vi "PH_Powermeter_BaseClass.ProcCases.vi"(0 "i ref in":refnum<vi>, 1 "selector":string, 2 "Data":T1, 3 "call cluster":T2={"Object"="", "Selector"="", "CallType"=enum."synchronous", "Async Object"="", "Async Selector"="", "Data Descriptor"="", "Data"=[], "Error #"=0, "Expire"=0}, 5 "error in":errorcluster) -> (14 "i ref out":refnum<vi>, 17 "answer cluster":T2={"Object"="", "Selector"="", "CallType"=enum."synchronous", "Async Object"="", "Async Selector"="", "Data Descriptor"="", "Data"=[], "Error #"=0, "Expire"=0}, 19 "error out":errorcluster)   [LabVIEW 2014, in "PH_Powermeter_BaseClass.lvlib"]
doc: "This method is called by a process from within the default case in the event loop. The methods of a class that are linked to events will be called from THIS method. Add your code here."
uses:
  PH_Powermeter_BaseClass.lvlib
  CS_Core/CSSystem/CoreDefs/CoreDefs.call_type.ctl
  CS_Core/BaseProcess/BaseProcess.descriptor string definition.ctl
  CS_Core/CSSystem/CoreDefs/CoreDefs.rawDataType.ctl
  CS_Core/CSSystem/CoreLib/CoreLib.string 2 byte array.vi
  CS_Core/CSSystem/CoreLib/CoreLib.byte array 2 int.vi
  CS_Core/CSSystem/CoreLib/CoreLib.byte array 2 double.vi
  CS_Core/CSSystem/CoreLib/CoreLib.lvlib
  CS_Core/BaseProcess/BaseProcess.lvlib
  PH_PSDBWriter/PH_PSDBWriter.lvlib
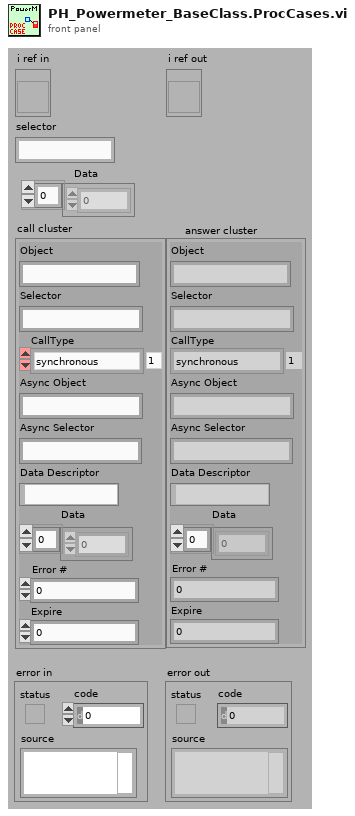
[diagram p1: front panel]
types:
  T1 = typedef "CoreDefs.rawDataType.ctl" = i8[]
  T2 = typedef "CoreDefs.call_type.ctl" = cluster{"Object":string, "Selector":string, "CallType":enum16{"simple", "synchronous", "asynchronous"}, "Async Object":string, "Async Selector":string, "Data Descriptor":T3, "Data":T1, "Error #":i32, "Expire":u32}
  T3 = typedef "BaseProcess.lvlib/BaseProcess.descriptor string definition.ctl" = string
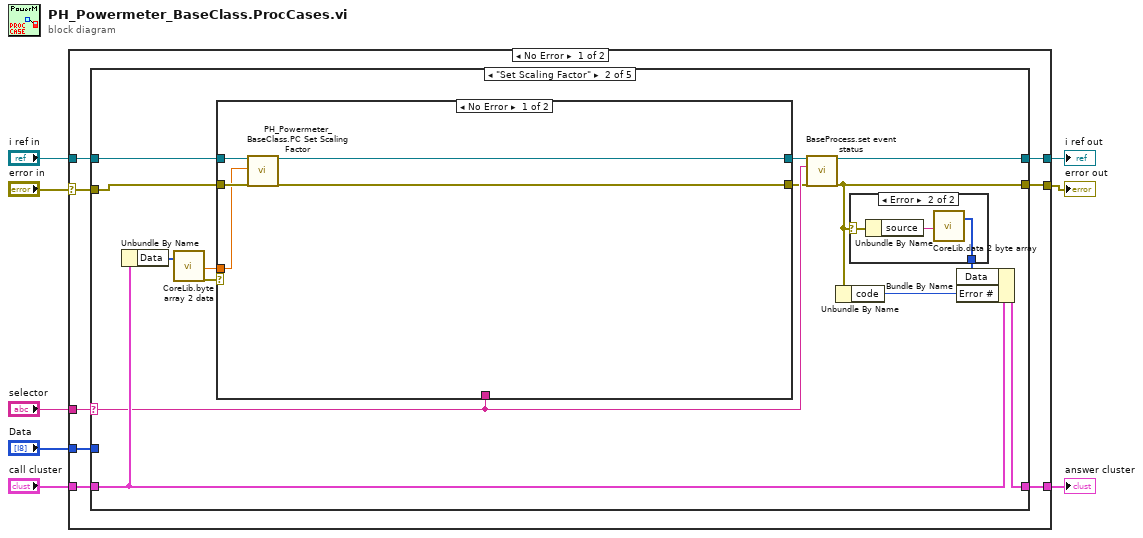
[diagram p0: block diagram]
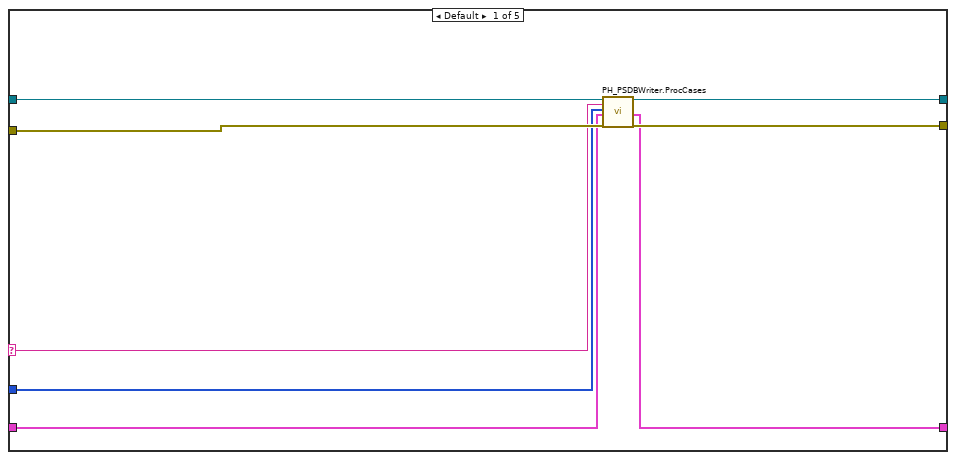
[diagram p2: hidden frame]
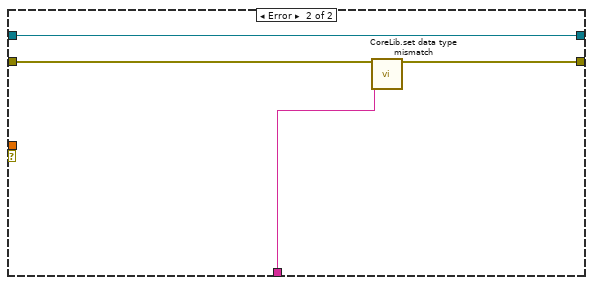
[diagram p4: hidden frame]
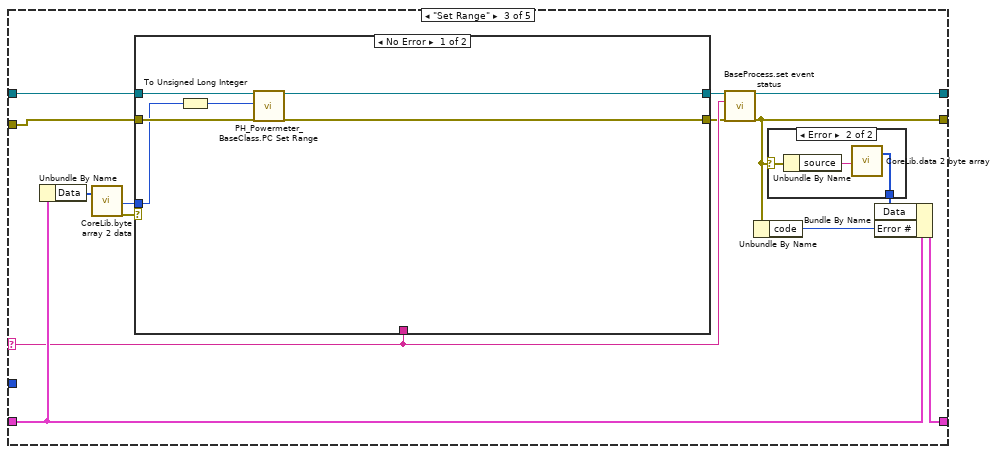
[diagram p5: hidden frame]
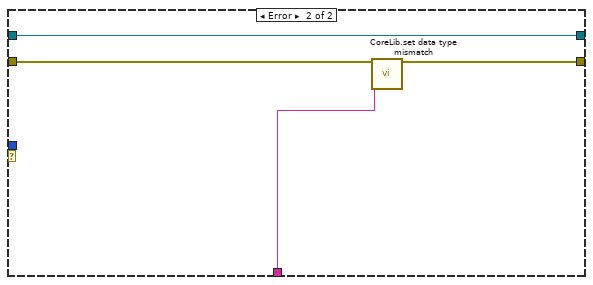
[diagram p7: hidden frame]
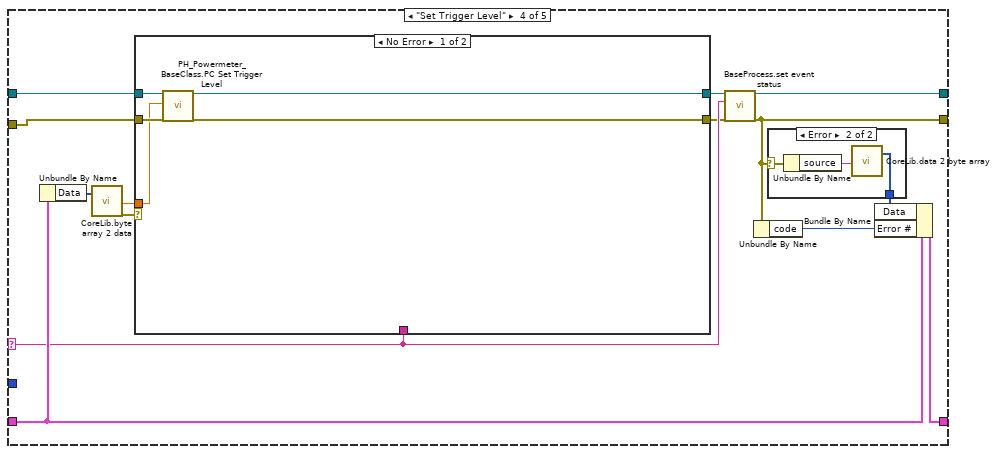
[diagram p8: hidden frame]
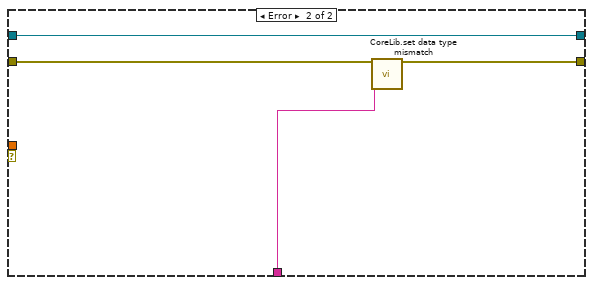
[diagram p10: hidden frame]
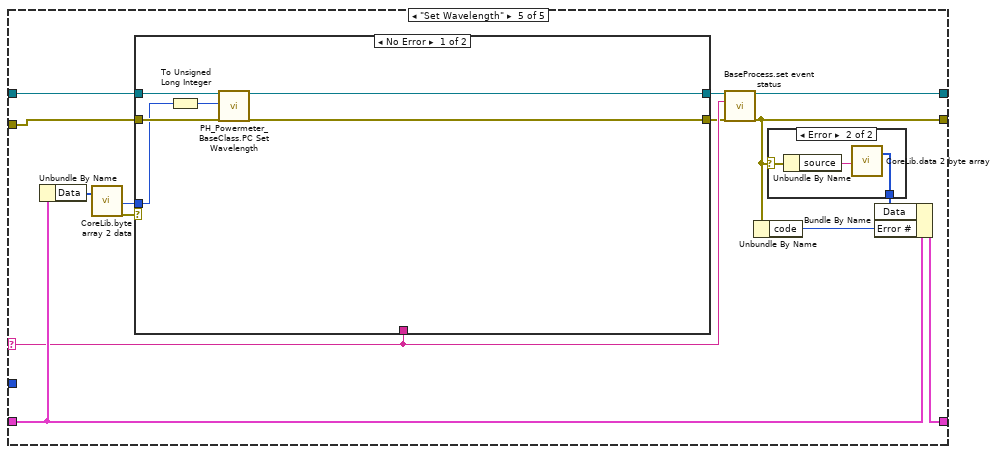
[diagram p11: hidden frame]
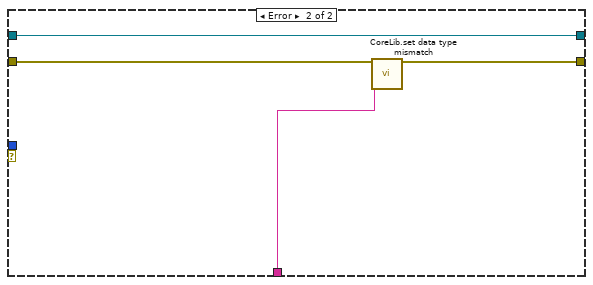
[diagram p13: hidden frame]
diagram:
  n1 = case shown="No Error" "error in" {
    selector: "error in" -> [w9 w132]
    tunnel: "selector" -> [w16 _]
    tunnel: [w15 w131] -> w7
    tunnel: "call cluster" -> [w14 w131]
    tunnel: "i ref in" -> [w13 w133]
    tunnel: [w12 w133] -> w4
    tunnel: [w11 w132] -> w1
    tunnel: "Data" -> [w10 _]
    frame No Error {
      n2 = case shown="\"Set Scaling Factor\"" w16 {
        selector: w16 -> [w19 w32 w58 w85 w111]
        tunnel: w13 -> [w18 w38 w64 w91 w117]
        tunnel: [w24 w33 w59 w86 w112] -> w12
        tunnel: w14 -> [w20 w35 w61 w88 w114]
        tunnel: [w21 w26 w52 w79 w105] -> w15
        tunnel: w9 -> [w23 w37 w63 w90 w116]
        tunnel: [w22 w34 w60 w87 w113] -> w11
        tunnel: w10 -> [w17 _ _ _ _]
        frame Default {
          # "In the default case, always call the ProcCase method of the parent class"
          n3 = call "PH_PSDBWriter.ProcCases.vi"("i ref in"=w18, "selector"=w19, "Data"=w17, "call cluster"=w20, "error in"=w23) -> ("i ref out"=w24:refnum<vi>, "answer cluster"=w21:T2, "error out"=w22:errorcluster)  [unwired: 12 in]
        }
        frame "Set Scaling Factor" {
          n4 = Unbundle By Name(w35) -> ("Data"=w29:T1)
          n5 = call-poly "CoreLib.byte array 2 data.vi"("byteArray"=w29) -> ("d64"=w28:dbl, "error out"=w27:errorcluster)  [unwired: 16 in, 1 out]
          n6 = case shown="No Error" w27 {
            tunnel: [w45 w50] -> w30
            tunnel: w38 -> [w46 w50]
            tunnel: w37 -> [w44 w49]
            tunnel: [w43 w48] -> w31
            tunnel: w32 -> [_ w47]
            tunnel: w28 -> [w42 _]
            frame No Error {
              n7 = call "PH_Powermeter_BaseClass.PC Set Scaling Factor.vi"("VI in"=w46, "Scaling Factor"=w42, "error in (no error)"=w44) -> ("VI out"=w45:refnum<vi>, "error out"=w43:errorcluster)  [unwired: 15 in]
            }
            frame Error {
              n8 = call "CoreLib.set data type mismatch.vi"("error in (no error)"=w49, "error source"=w47) -> ("error out"=w48:errorcluster)  [unwired: 17 in]
            }
          }
          n9 = call "BaseProcess.set event status.vi"("i ref in"=w30, "EventStatus"=w32, "error in (no error)"=w31) -> ("i ref out"=w33:refnum<vi>, "error out"=w34:errorcluster)  [unwired: 14 in, 1 out]
          n10 = Unbundle By Name(w34) -> ("code"=w36:i32)
          n11 = case shown="Error" w34 {
            selector: w34 -> [_ w41]
            tunnel: [_ w39] -> w25
            frame No Error {
            }
            frame Error {
              n12 = Unbundle By Name(w41) -> ("source"=w40:string)
              n13 = call-poly "CoreLib.data 2 byte array.vi"("string"=w40) -> ("byteArray out"=w39:T1)  [unwired: 18 in]
            }
          }
          n14 = Bundle By Name(cluster=w35, "Data"=w25, "Error #"=w36) -> (w26:T2)
        }
        frame "Set Range" {
          n15 = Unbundle By Name(w61) -> ("Data"=w55:T1)
          n16 = call-poly "CoreLib.byte array 2 data.vi"("byteArray"=w55) -> ("i32"=w54:i32, "error out"=w53:errorcluster)  [unwired: 16 in, 1 out]
          n17 = case shown="No Error" w53 {
            tunnel: [w72 w77] -> w56
            tunnel: w64 -> [w73 w77]
            tunnel: w63 -> [w71 w76]
            tunnel: [w70 w75] -> w57
            tunnel: w58 -> [_ w74]
            tunnel: w54 -> [w69 _]
            frame No Error {
              n18 = To Unsigned Long Integer(number=w69) -> (unsigned 32bit integer=w68:u32)
              n19 = call "PH_Powermeter_BaseClass.PC Set Range.vi"("VI in"=w73, "Wanted Range"=w68, "error in (no error)"=w71) -> ("VI out"=w72:refnum<vi>, "error out"=w70:errorcluster)  [unwired: 15 in]
            }
            frame Error {
              n20 = call "CoreLib.set data type mismatch.vi"("error in (no error)"=w76, "error source"=w74) -> ("error out"=w75:errorcluster)  [unwired: 17 in]
            }
          }
          n21 = call "BaseProcess.set event status.vi"("i ref in"=w56, "EventStatus"=w58, "error in (no error)"=w57) -> ("i ref out"=w59:refnum<vi>, "error out"=w60:errorcluster)  [unwired: 14 in, 1 out]
          n22 = Unbundle By Name(w60) -> ("code"=w62:i32)
          n23 = case shown="Error" w60 {
            selector: w60 -> [_ w67]
            tunnel: [_ w65] -> w51
            frame No Error {
            }
            frame Error {
              n24 = Unbundle By Name(w67) -> ("source"=w66:string)
              n25 = call-poly "CoreLib.data 2 byte array.vi"("string"=w66) -> ("byteArray out"=w65:T1)  [unwired: 18 in]
            }
          }
          n26 = Bundle By Name(cluster=w61, "Data"=w51, "Error #"=w62) -> (w52:T2)
        }
        frame "Set Trigger Level" {
          n27 = Unbundle By Name(w88) -> ("Data"=w82:T1)
          n28 = call-poly "CoreLib.byte array 2 data.vi"("byteArray"=w82) -> ("d64"=w81:dbl, "error out"=w80:errorcluster)  [unwired: 16 in, 1 out]
          n29 = case shown="No Error" w80 {
            tunnel: [w98 w103] -> w83
            tunnel: w91 -> [w99 w103]
            tunnel: w90 -> [w97 w102]
            tunnel: [w96 w101] -> w84
            tunnel: w85 -> [_ w100]
            tunnel: w81 -> [w95 _]
            frame No Error {
              n30 = call "PH_Powermeter_BaseClass.PC Set Trigger Level.vi"("VI in"=w99, "Wanted Trigger Level [%]"=w95, "error in (no error)"=w97) -> ("VI out"=w98:refnum<vi>, "error out"=w96:errorcluster)  [unwired: 15 in]
            }
            frame Error {
              n31 = call "CoreLib.set data type mismatch.vi"("error in (no error)"=w102, "error source"=w100) -> ("error out"=w101:errorcluster)  [unwired: 17 in]
            }
          }
          n32 = call "BaseProcess.set event status.vi"("i ref in"=w83, "EventStatus"=w85, "error in (no error)"=w84) -> ("i ref out"=w86:refnum<vi>, "error out"=w87:errorcluster)  [unwired: 14 in, 1 out]
          n33 = Unbundle By Name(w87) -> ("code"=w89:i32)
          n34 = case shown="Error" w87 {
            selector: w87 -> [_ w94]
            tunnel: [_ w92] -> w78
            frame No Error {
            }
            frame Error {
              n35 = Unbundle By Name(w94) -> ("source"=w93:string)
              n36 = call-poly "CoreLib.data 2 byte array.vi"("string"=w93) -> ("byteArray out"=w92:T1)  [unwired: 18 in]
            }
          }
          n37 = Bundle By Name(cluster=w88, "Data"=w78, "Error #"=w89) -> (w79:T2)
        }
        frame "Set Wavelength" {
          n38 = Unbundle By Name(w114) -> ("Data"=w108:T1)
          n39 = call-poly "CoreLib.byte array 2 data.vi"("byteArray"=w108) -> ("i32"=w107:i32, "error out"=w106:errorcluster)  [unwired: 16 in, 1 out]
          n40 = case shown="No Error" w106 {
            tunnel: [w125 w130] -> w109
            tunnel: w117 -> [w126 w130]
            tunnel: w116 -> [w124 w129]
            tunnel: [w123 w128] -> w110
            tunnel: w111 -> [_ w127]
            tunnel: w107 -> [w122 _]
            frame No Error {
              n41 = To Unsigned Long Integer(number=w122) -> (unsigned 32bit integer=w121:u32)
              n42 = call "PH_Powermeter_BaseClass.PC Set Wavelength.vi"("VI in"=w126, "Wanted Wavelength [nm]"=w121, "error in (no error)"=w124) -> ("VI out"=w125:refnum<vi>, "error out"=w123:errorcluster)  [unwired: 15 in]
            }
            frame Error {
              n43 = call "CoreLib.set data type mismatch.vi"("error in (no error)"=w129, "error source"=w127) -> ("error out"=w128:errorcluster)  [unwired: 17 in]
            }
          }
          n44 = call "BaseProcess.set event status.vi"("i ref in"=w109, "EventStatus"=w111, "error in (no error)"=w110) -> ("i ref out"=w112:refnum<vi>, "error out"=w113:errorcluster)  [unwired: 14 in, 1 out]
          n45 = Unbundle By Name(w113) -> ("code"=w115:i32)
          n46 = case shown="Error" w113 {
            selector: w113 -> [_ w120]
            tunnel: [_ w118] -> w104
            frame No Error {
            }
            frame Error {
              n47 = Unbundle By Name(w120) -> ("source"=w119:string)
              n48 = call-poly "CoreLib.data 2 byte array.vi"("string"=w119) -> ("byteArray out"=w118:T1)  [unwired: 18 in]
            }
          }
          n49 = Bundle By Name(cluster=w114, "Data"=w104, "Error #"=w115) -> (w105:T2)
        }
      }
    }
    frame Error {
    }
  }
  "answer cluster" <- w7
  "i ref out" <- w4
  "error out" <- w1
